vi "Waveform to ns timestamp.vi"(11 "Waveform":waveform(dbl)) -> (1 "number of samples":i32, 2 "data":dbl[](array[numeric]), 3 "ns timestamp":u64[](array[numeric]))   [LabVIEW 2020, in "Nominal Streaming.lvlib"]
uses:
  Nominal Streaming.lvlib
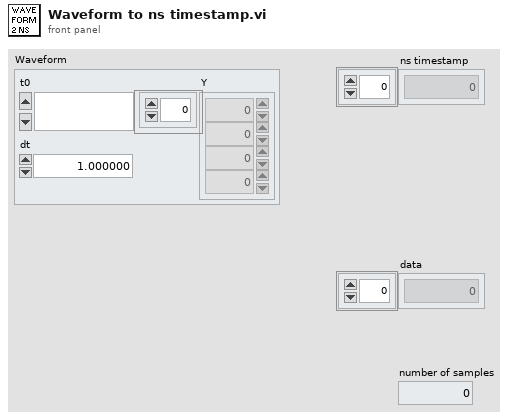
[diagram p1: front panel]
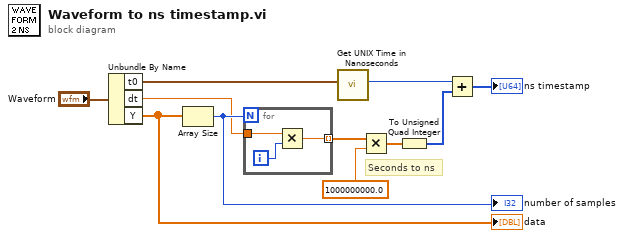
[diagram p0: block diagram]
diagram:
  # "Seconds to ns"
  n1 = Unbundle By Name("Waveform") -> ("t0"=w10:timestamp, "dt"=w7:dbl, "Y"=w11:dbl[])
  "data" <- w11
  n2 = Array Size(array=w11) -> (size(s)=w8:i32)
  "number of samples" <- w8
  n3 = for {
    N: w8 -> [_]
    tunnel: w7 -> [w13]
    tunnel: [w12] -> w6 mode=indexing
    i -> [w14]
    n4 = Multiply(x=w13, y=w14) -> (x*y=w12:dbl)
  }
  n5 = call "Get UNIX Time in Nanoseconds.vi"("Time Stamp"=w10) -> ("UNIX Time (ns)"=w3:u64)  [unwired: 10 in]
  n6 = Multiply(x=w6, y=1000000000.0 ("dt")) -> (x*y=w4:dbl[])
  n7 = To Unsigned Quad Integer(1:w4) -> (0:w2:u64[])
  n8 = Add(x=w3, y=w2) -> (x+y=→"ns timestamp":u64[])
